vi "Reset.vi"(8 "Error In (no error)":errorcluster, 9 "Delay After Reset (2000 ms)":u32=2000, 10 "Motor ID (0)":u8, 11 "VISA resource name":refnum<visa-resource-name>) -> (0 "error out":errorcluster, 3 "VISA resource name out":refnum<visa-resource-name>)   [LabVIEW 2016, in "Dynamixel Motor.lvlib"]
doc: "Resets the motor and to its default values. The motor ID will be 1 and the baud rate will be 57600 bps."
uses:
  Dynamixel Motor.lvlib
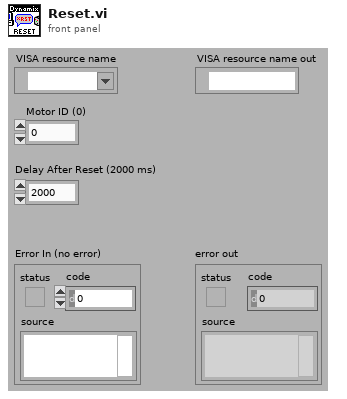
[diagram p1: front panel]
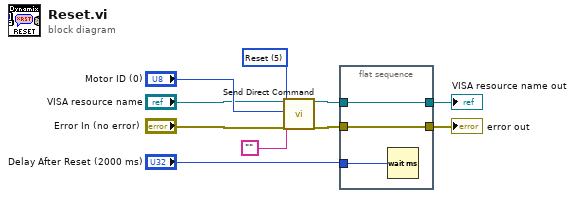
[diagram p0: block diagram]
diagram:
  w7 = u16 5 items=["Ping", "Read", "Write", "Registered Write", "Action", "Reset", "Sync Write"] ("Select Action")
  n1 = call "Send Direct Command.vi"("VISA resource name"="VISA resource name", "Select Action"=w7, "Motor ID (0)"="Motor ID (0)", "Parameters"="", "Error in (no error)"="Error In (no error)") -> ("VISA resource name out"=w2:refnum<visa-resource-name>, "Error out"=w4:errorcluster)  [unwired: 12 in, 1 out]
  n2 = flat-sequence {
    tunnel: "Delay After Reset (2000 ms)" -> [w13]
    tunnel: w4 -> [w12]
    tunnel: [w12] -> w3
    tunnel: w2 -> [w11]
    tunnel: [w11] -> w1
    frame #0 {
      n3 = Wait (ms)(milliseconds to wait=w13) -> ()  [unwired: 1 out]
    }
  }
  "error out" <- w3
  "VISA resource name out" <- w1
